vi "Example v2.vi"() -> ()   [LabVIEW 2020, in "Arduino.lvlib"]
doc: "This example performs writes and reads on a serial port, as directed by the user. You can press the Write and Read buttons, and change the Read Count, while the example is running.\n\nThe parameters set for the serial port must match the parameters of the connected instrument or device. In this example, the Read Count parameter specifies the number of bytes that the serial port reads. If there were more bytes at the port than the specified number, those bytes would not be read. If there were less bytes at the port than the specified number, you would receive a timeout error.\n\nThis example expands upon the flow control options for XON and XOFF, allowing the user to choose those control characters. Also, the user can enable or disable a termination character. Some devices require a termination character in order to identify the end of command strings. Some devices send a termination character to signify the end of data to be read. This example shows how you can end the Read operation once a termination character is detected in the buffer and/or append a termination character at the end of the Write data."
uses:
  Arduino.lvlib
  <vilib>/National Instruments/Variant Ring Buffer/Ring Buffer.lvclass
  Arduino.lvclass
panel:
  in  "write":bool
  out "Response":string="519 \t519 \t518 \t518 \t518 \t518 \t518 \t519 \t518 \t518\t1023 \t1023 \t1023 \t1023 \t1023 \t1023 \t1023 \t1023 \t1023 \t1023\t45 \t45 \t45 \t45 \t46 \t45 \t46 \t45 \t46 \t46\t63 \t63 \t63 \t62 \t63 \t63 \t62 \t63 \t62 \t63\t0 \t1 \t0 \t1 \t0 \t1 \t0 \t0 \t1 \t1\t0 \t0 \t1 \t0 \t1 \t1 \t1 \t0 \t1 \t0\t\r\n"
  in  "Serial Settings":T1={"baud rate"=115200, "data bits"=8, "parity"=enum."None", "stop bits"=10, "flow control"=0} {"flow control" items=["None"=0, "XON/XOFF"=1, "RTS/CTS"=2, "DTR/DSR"=4]; "stop bits" items=["1.0"=10, "1.5"=15, "2.0"=20]; "data bits" min=5 max=8 step=1; "baud rate" items=["75"=75, "110"=110, "134"=134, "150"=150, "300"=300, "600"=600, "1200"=1200, "1800"=1800, "2400"=2400, "4800"=4800, "7200"=7200, "9600"=9600, "14400"=14400, "19200"=19200, "28800"=28800, "38400"=38400, "56000"=56000, "57600"=57600, "115200"=115200, "128000"=128000, "230400"=230400]}
  in  "VISA":refnum<visa-resource-name>="COM3"
  out "Chart":dbl[][](graph)
  out "Number of Bytes at Serial Port":u32=246
  in  "Stop":bool
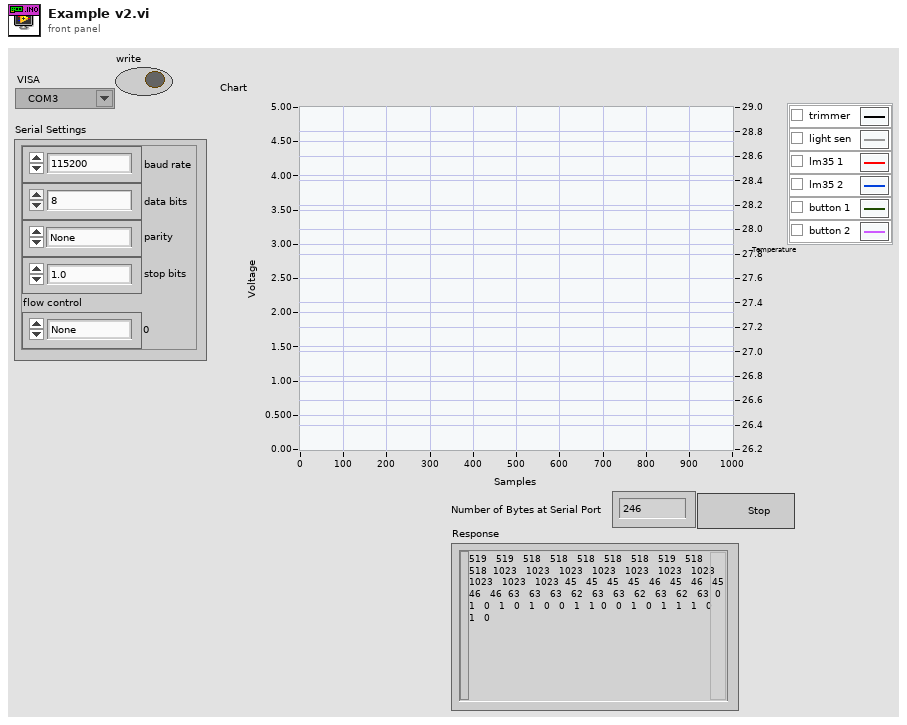
[diagram p1: front panel]
types:
  T1 = cluster{"baud rate":u32, "data bits":u16, "parity":enum16{"None", "Odd", "Even", "Mark", "Space"}, "stop bits":u16, "flow control":u16}
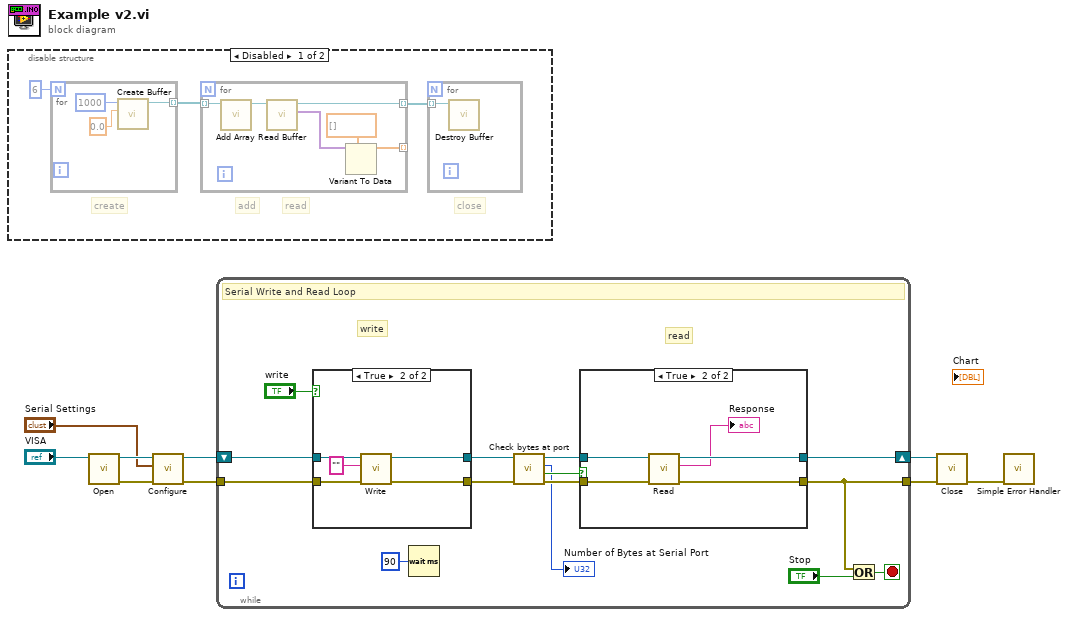
[diagram p0: block diagram]
diagram:
  n1 = disable-structure shown="Disabled" {
    frame Disabled {
      # "close"
      # "read"
      # "add"
      # "create"
      n2 = for {
        N: 6 -> [_]
        tunnel: [w20] -> w11 mode=indexing
        n3 = call <vilib>:"Create Buffer.vi"("Data Type"=0.0, "Buffer Size"=1000) -> ("Ring Buffer Reference"=w20:refnum<data-value>)  [unwired: 8 in, 1 out]
      }
      n4 = for {
        tunnel: w11 -> [w19] mode=indexing
        tunnel: [w17] -> w10 mode=indexing
        tunnel: [w14] -> _ mode=indexing
        n5 = call <vilib>:"Add Array.vi"("Ring Buffer Reference"=w19) -> ("Ring Buffer Reference"=w18:refnum<data-value>)  [unwired: 9 in, 1 out]
        n6 = call <vilib>:"Read Buffer.vi"("Ring Buffer Reference"=w18) -> ("Array of Variants"=w16:variant[], "Ring Buffer Reference"=w17:refnum<data-value>)  [unwired: 8 in, 1 out]
        n7 = Variant To Data(type=dbl[] [] ("subarray"), Variant=w16) -> (data=w14:dbl[])  [unwired: 1 in, 1 out]
      }
      n8 = for {
        tunnel: w10 -> [w13] mode=indexing
        n9 = call <vilib>:"Destroy Buffer.vi"("Ring Buffer Reference"=w13) -> ()  [unwired: 9 in, 2 out]
      }
    }
    frame Enabled {
    }
  }
  n10 = call "Open.vi"("VISA"="VISA") -> ("error out"=w5:errorcluster, "ArduinoAIReal out"=w6:refnum<class "Arduino.lvclass">)  [unwired: 9 in]
  n11 = call "Configure.vi"("error in (no error)"=w5, "Serial Settings"="Serial Settings", "ArduinoAIReal in"=w6) -> ("error out"=w2:errorcluster, "ArduinoAIReal out"=w3:refnum<class "Arduino.lvclass">)  [unwired: 7 in]
  n12 = while {
    shift-right: [w28] -> w9
    shift-left: w3 -> [w27]
    tunnel: [w34] -> w7
    tunnel: w2 -> [w24]
    stop <- w35 stop-if-true
    # "read"
    # "write"
    # "Serial Write and Read Loop"
    n13 = case shown="True" "write" {
      tunnel: w27 -> [w38 w43]
      tunnel: [w38 w42] -> w26
      tunnel: [w37 w41] -> w25
      tunnel: w24 -> [w37 w40]
      frame False {
      }
      frame True {
        n14 = call "Write.vi"("error in (no error)"=w40, "write buffer"="", "ArduinoAIReal in"=w43) -> ("error out"=w41:errorcluster, "ArduinoAIReal out"=w42:refnum<class "Arduino.lvclass">)  [unwired: 7 in]
      }
    }
    n15 = Wait (ms)(milliseconds to wait=u32 90) -> ()  [unwired: 1 out]
    n16 = call "Check bytes at port.vi"("error in (no error)"=w25, "ArduinoAIReal in"=w26) -> ("error out"=w31:errorcluster, "Bytes available"=w32:bool, "Number of Bytes at Serial Port"=→"Number of Bytes at Serial Port":u32, "ArduinoAIReal out"=w29:refnum<class "Arduino.lvclass">)  [unwired: 6 in]
    n17 = case shown="True" w32 {
      tunnel: [w45 w48] -> w28
      tunnel: [w44 w47] -> w34
      tunnel: w31 -> [w44 w49]
      tunnel: w29 -> [w45 w50]
      frame False {
      }
      frame True {
        n18 = call "Read.vi"("error in (no error)"=w49, "ArduinoAIReal in"=w50) -> ("error out"=w47:errorcluster, "Response"=→"Response":string, "ArduinoAIReal out"=w48:refnum<class "Arduino.lvclass">)  [unwired: 7 in]
      }
    }
    n19 = Or(x=w34, y="Stop") -> (x .or. y?=w35:bool)
  }
  n20 = call "Close.vi"("error in (no error)"=w7, "ArduinoAIReal in"=w9) -> ("error out"=w8:errorcluster)  [unwired: 9 in]
  n21 = call <vilib>:"Simple Error Handler.vi"("error in (no error)"=w8) -> ()  [unwired: 1 in, 8 out]
